vi "If The Position is in List.vi"(9 "column":i32, 10 "row":i32, 11 "available position":i32[][](array[numeric])) -> (1 "found?":bool)   [LabVIEW 2011, in "Othello.xctl"]
uses:
  Othello.xctl
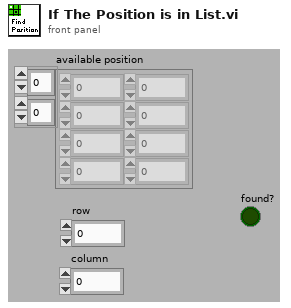
[diagram p1: front panel]
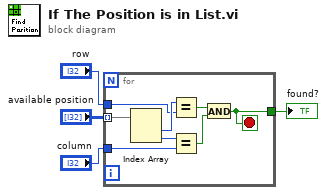
[diagram p0: block diagram]
diagram:
  n1 = for {
    tunnel: "available position" -> [w12] mode=indexing
    tunnel: "row" -> [w10]
    tunnel: "column" -> [w8]
    tunnel: [w5] -> w1
    stop <- w5 stop-if-true
    n2 = Index Array(array=w12) -> (element #1=w11:i32, element #2=w9:i32)  [unwired: 2 in]
    n3 = Equal?(x=w11, y=w10) -> (x = y?=w7:bool)
    n4 = Equal?(x=w9, y=w8) -> (x = y?=w6:bool)
    n5 = And(x=w7, y=w6) -> (x .and. y?=w5:bool)
  }
  "found?" <- w1
